vi "Write Setting.vi"(0 "configuration file path":path, 1 "output cluster":T1, 3 "error in (no error)":errorcluster) -> (7 "file path":path, 10 "error out":errorcluster)   [LabVIEW 2023]
uses:
  <vilib>/Utility/config.llb/Write Key (String).vi
  <vilib>/Utility/config.llb/Write Key (U32).vi
  <vilib>/Utility/config.llb/Write Key (I32).vi
  <vilib>/Utility/config.llb/Write Key (Double).vi
  <vilib>/Utility/config.llb/Write Key (Path).vi
  <vilib>/Utility/config.llb/NI_LVConfig.lvlib
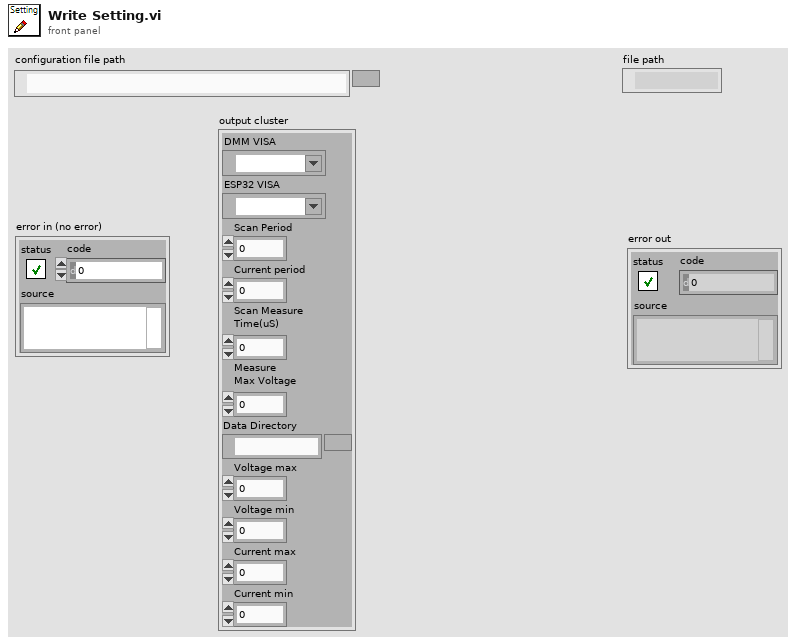
[diagram p1: front panel]
types:
  T1 = cluster{"DMM VISA":refnum<visa-resource-name>, "ESP32 VISA":refnum<visa-resource-name>, "Scan Period":u32, "Current period":u32, "Scan Measure\nTime(uS)":i32, "Measure\nMax Voltage":dbl, "Data Directory":path, "Voltage max":dbl, "Voltage min":dbl, "Current max":dbl, "Current min":dbl}
  T2 = typedef "NI_LVConfig.lvlib/Config Data RefNum.ctl" = refnum<k1>
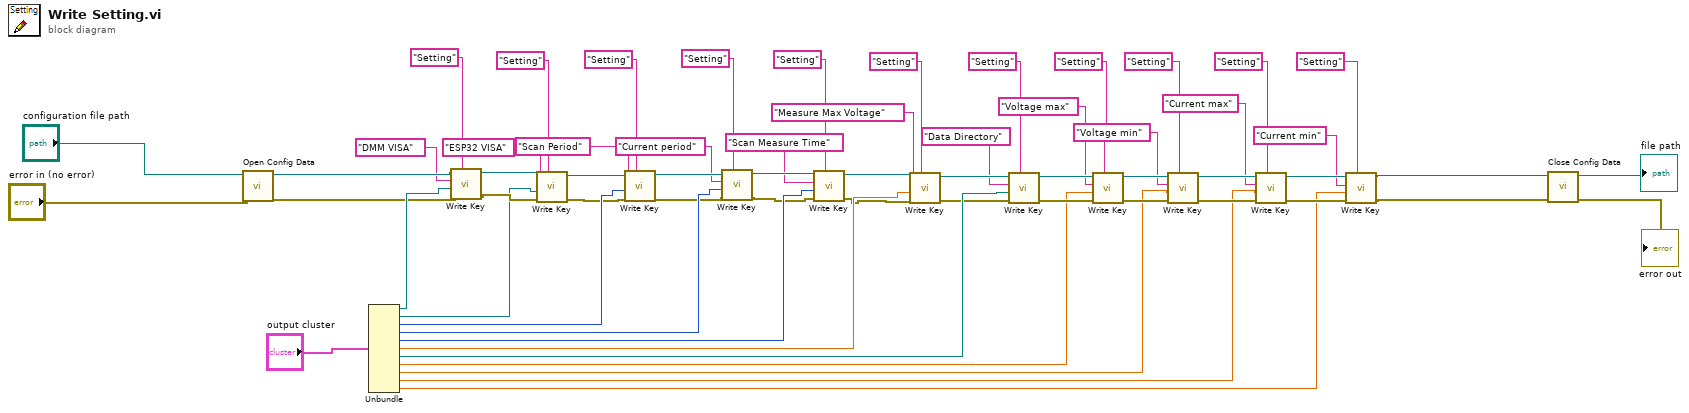
[diagram p0: block diagram]
diagram:
  n1 = call <vilib>:"Open Config Data.vi"("error in (no error)"="error in (no error)", "configuration file path"="configuration file path") -> ("error out"=w44:errorcluster, "refnum"=w45:T2)  [unwired: 7 in, 1 out]
  n2 = Unbundle("output cluster") -> ("DMM VISA"=w57:refnum<visa-resource-name>, "ESP32 VISA"=w30:refnum<visa-resource-name>, "Scan Period"=w51:u32, "Current period"=w50:u32, "Scan Measure\nTime(uS)"=w49:i32, "Measure\nMax Voltage"=w48:dbl, "Data Directory"=w46:path, "Voltage max"=w10:dbl, "Voltage min"=w9:dbl, "Current max"=w8:dbl, "Current min"=w7:dbl)
  n3 = call-poly <vilib>:"Write Key.vi"("section"="Setting", "error in (no error)"=w44, "value"=w57, "key"="DMM VISA", "refnum"=w45) -> ("error out"=w32:errorcluster, "refnum out"=w43:T2)  [unwired: 4 in, 1 out]
  n4 = call-poly <vilib>:"Write Key.vi"("section"="Setting", "error in (no error)"=w32, "value"=w30, "key"="ESP32 VISA", "refnum"=w43) -> ("error out"=w41:errorcluster, "refnum out"=w42:T2)  [unwired: 4 in, 1 out]
  n5 = call-poly <vilib>:"Write Key.vi"("section"="Setting", "error in (no error)"=w41, "value"=w51, "key"="Scan Period", "refnum"=w42) -> ("error out"=w39:errorcluster, "refnum out"=w40:T2)  [unwired: 4 in, 1 out]
  n6 = call-poly <vilib>:"Write Key.vi"("section"="Setting", "error in (no error)"=w39, "value"=w50, "key"="Current period", "refnum"=w40) -> ("error out"=w37:errorcluster, "refnum out"=w38:T2)  [unwired: 4 in, 1 out]
  n7 = call-poly <vilib>:"Write Key.vi"("section"="Setting", "error in (no error)"=w37, "value"=w49, "key"="Scan Measure Time", "refnum"=w38) -> ("error out"=w35:errorcluster, "refnum out"=w36:T2)  [unwired: 4 in, 1 out]
  n8 = call-poly <vilib>:"Write Key.vi"("section"="Setting", "error in (no error)"=w35, "value"=w48, "key"="Measure Max Voltage", "refnum"=w36) -> ("error out"=w33:errorcluster, "refnum out"=w34:T2)  [unwired: 4 in, 1 out]
  n9 = call-poly <vilib>:"Write Key.vi"("section"="Setting", "error in (no error)"=w33, "value"=w46, "key"="Data Directory", "refnum"=w34) -> ("error out"=w23:errorcluster, "refnum out"=w16:T2)  [unwired: 4 in, 1 out]
  n10 = call-poly <vilib>:"Write Key.vi"("section"="Setting", "error in (no error)"=w23, "value"=w10, "key"="Voltage max", "refnum"=w16) -> ("error out"=w21:errorcluster, "refnum out"=w22:T2)  [unwired: 4 in, 1 out]
  n11 = call-poly <vilib>:"Write Key.vi"("section"="Setting", "error in (no error)"=w21, "value"=w9, "key"="Voltage min", "refnum"=w22) -> ("error out"=w19:errorcluster, "refnum out"=w20:T2)  [unwired: 4 in, 1 out]
  n12 = call-poly <vilib>:"Write Key.vi"("section"="Setting", "error in (no error)"=w19, "value"=w8, "key"="Current max", "refnum"=w20) -> ("error out"=w17:errorcluster, "refnum out"=w18:T2)  [unwired: 4 in, 1 out]
  n13 = call-poly <vilib>:"Write Key.vi"("section"="Setting", "error in (no error)"=w17, "value"=w7, "key"="Current min", "refnum"=w18) -> ("error out"=w1:errorcluster, "refnum out"=w2:T2)  [unwired: 4 in, 1 out]
  n14 = call <vilib>:"Close Config Data.vi"("error in (no error)"=w1, "refnum"=w2) -> ("error out"=→"error out":errorcluster, "file path"=→"file path":path)  [unwired: 8 in]
